vi "Parse Measurement Data.vi"(8 "error in (no error)":errorcluster, 10 "Measurement Parameters":T1={"Start Step"=44, "End Step"=725, "Cluster Count"=1, "Scan Interval"=0, "Number of Scans"=0, "Measurement Type"=enum."MS"}, 11 "VISA Refnum in":refnum<visa-resource-name>) -> (0 "error out":errorcluster, 2 "Measurement Data":i32[](array[numeric]), 3 "VISA Refnum out":refnum<visa-resource-name>)   [LabVIEW 2016]
doc: "Reads a measurement packet from the URG-04LX. This will only return data if an acquisition has been started."
uses:
  Type Definitions/Controls/Measurement Parameters.ctl
  Type Definitions/Controls/Measurement Type.ctl
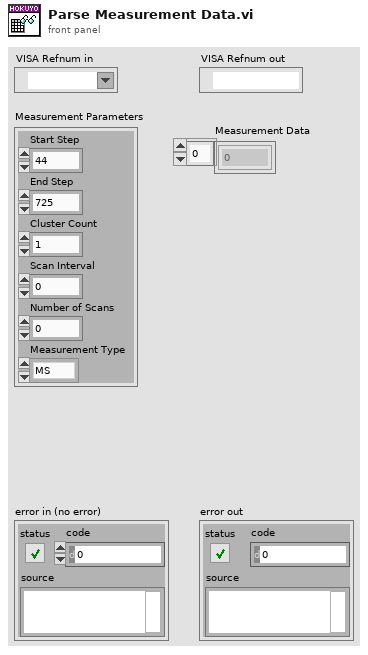
[diagram p1: front panel]
types:
  T1 = typedef "Measurement Parameters.ctl" = cluster{"Start Step":u32, "End Step":u32, "Cluster Count":u32, "Scan Interval":u32, "Number of Scans":u32, "Measurement Type":T2}
  T2 = typedef "Measurement Type.ctl" = enum16{"MS"}
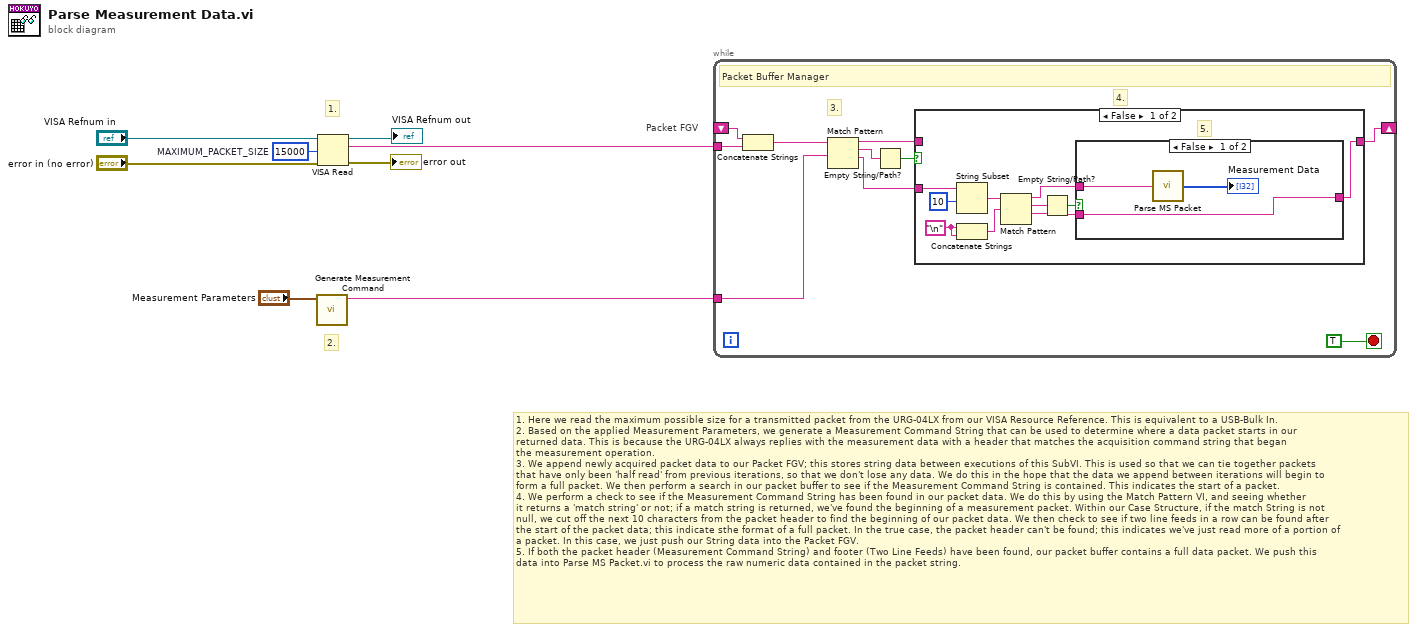
[diagram p0: block diagram]
diagram:
  w8 = u32 15000  # MAXIMUM_PACKET_SIZE
  # "Packet FGV"
  # "1. Here we read the maximum possible size for a transmitted packet from the URG-04LX from our VISA Resource Reference. This is equivalent to a USB-Bulk In.\n2. Based on the applied Measurement Parameters, we generate a Measurement Command String that can be used to determine where a data packet starts in our\nreturned data. This is because the URG-04LX always replies with the measurement data with a header that matches the acquisition command string that began \nthe measurement operation.\n3. We append newly acquired packet data to our Packet FGV; this stores string data between executions of this SubVI. This is used so that we can tie together packets\nthat have only been 'half read' from previous iterations, so that we don't lose any data. We do this in the hope that the data we append between iterations will begin to\nform a full packet. We then perform a search in our packet buffer to see if the Measurement Command String is contained. This indicates the start of a packet.\n4. We perform a check to see if the Measurement Command String has been found in our packet data. We do this by using the Match Pattern VI, and seeing whether\nit returns a 'match string' or not; if a match string is returned, we've found the beginning of a measurement packet. Within our Case Structure, if the match String is not\nnull, we cut off the next 10 characters from the packet header to find the beginning of our packet data. We then check to see if two line feeds in a row can be found after\nthe start of the packet data; this indicate sthe format of a full packet. In the true case, the packet header can't be found; this indicates we've just read more of a portion of \na packet. In this case, we just push our String data into the Packet FGV.\n5. If both the packet header (Measurement Command String) and footer (Two Line Feeds) have been found, our packet buffer contains a full data packet. We push this\ndata into Parse MS Packet.vi to process the raw numeric data contained in the packet string."
  # "2."
  # "1."
  n1 = call "Generate Measurement Command.vi"("Measurement Parameters"="Measurement Parameters") -> ("Measurement Command"=w2:string)  [unwired: 10 in]
  n2 = VISA Read(VISA resource name="VISA Refnum in", byte count=w8, error in (no error)="error in (no error)") -> (VISA resource name out=→"VISA Refnum out":refnum<visa-resource-name>, read buffer=w3:string, error out=→"error out":errorcluster)  [unwired: 1 out]
  n3 = while {
    tunnel: w3 -> [w16]
    tunnel: w2 -> [w9]
    shift-right: [w18] -> _
    shift-left: _ -> [w17]
    stop <- TRUE stop-if-true
    # "4."
    # "3."
    # "Packet Buffer Manager"
    n4 = Concatenate Strings(w17, w16) -> (w15:string)
    n5 = Match Pattern(string=w15, regular expression=w9) -> (before substring=w10:string, match substring=w13:string, after substring=w12:string)  [unwired: 1 in, 1 out]
    n6 = Empty String/Path?(string/path=w13) -> (empty?=w11:bool)
    n7 = case shown="False" w11 {
      tunnel: w12 -> [w24 _]
      tunnel: w10 -> [_ w33]
      tunnel: [w21 w33] -> w18
      frame False {
        w19 = "\n"
        # "5."
        n8 = String Subset(string=w24, offset (0)=10) -> (substring=w26:string)  [unwired: 1 in]
        n9 = Concatenate Strings(w19, w19) -> (w27:string)
        n10 = Match Pattern(string=w26, regular expression=w27) -> (before substring=w22:string, match substring=w28:string, after substring=w20:string)  [unwired: 1 in, 1 out]
        n11 = Empty String/Path?(string/path=w28) -> (empty?=w23:bool)
        n12 = case shown="False" w23 {
          tunnel: w22 -> [w30 w32]
          tunnel: [w31 w32] -> w21
          tunnel: w20 -> [w31 _]
          frame False {
            n13 = call "Parse MS Packet.vi"("Packet Measurement Data"=w30) -> ("Raw Height Data"=→"Measurement Data":i32[])
          }
          frame True {
          }
        }
      }
      frame True {
      }
    }
  }
